vi "test_heading_calculate.vi"() -> ()   [LabVIEW 2019]
panel:
  out "new picture":picture
  out "웨이브폼 차트":dbl(graph)
  out "숫자형":i32
  in  "dt":u32=100
  in  "정지":bool
  out "UTM graph":cluster{"X":dbl, "Y":dbl}[](graph)=[{"X"=3513.14928, "Y"=12901.22133}, {"X"=3513.14928, "Y"=12901.22136}, {"X"=3513.14928, "Y"=12901.22138}, {"X"=3513.14928, "Y"=12901.2214}, {"X"=3513.14928, "Y"=12901.22142}, {"X"=3513.14928, "Y"=12901.22144}, {"X"=3513.14928, "Y"=12901.22146}, {"X"=3513.14928, "Y"=12901.22149}, {"X"=3513.14928, "Y"=12901.2215}, {"X"=3513.14926, "Y"=12901.22148}, {"X"=3513.14917, "Y"=12901.22128}, {"X"=3513.14898, "Y"=12901.22091}, {"X"=3513.14873, "Y"=12901.22045}, {"X"=3513.14844, "Y"=12901.21994}, {"X"=3513.1481, "Y"=12901.21938}, {"X"=3513.14771, "Y"=12901.21876}, {"X"=3513.14726, "Y"=12901.21808}, {"X"=3513.14671, "Y"=12901.21736}, {"X"=3513.14601, "Y"=12901.21655}, {"X"=3513.14519, "Y"=12901.21573}, {"X"=3513.14431, "Y"=12901.21489}, {"X"=3513.14358, "Y"=12901.21391}, {"X"=3513.14334, "Y"=12901.21266}, {"X"=3513.14367, "Y"=12901.21139}, {"X"=3513.14447, "Y"=12901.21041}, {"X"=3513.14553, "Y"=12901.20996}, {"X"=3513.14662, "Y"=12901.21019}, {"X"=3513.14749, "Y"=12901.21113}, {"X"=3513.14818, "Y"=12901.21232}, {"X"=3513.14884, "Y"=12901.21355}, {"X"=3513.14951, "Y"=12901.21476}, {"X"=3513.15018, "Y"=12901.21596}, {"X"=3513.15082, "Y"=12901.21716}, {"X"=3513.15145, "Y"=12901.21839}, {"X"=3513.15204, "Y"=12901.2196}, {"X"=3513.15259, "Y"=12901.22082}, {"X"=3513.15311, "Y"=12901.22201}, {"X"=3513.15351, "Y"=12901.22323}, {"X"=3513.15362, "Y"=12901.2244}, {"X"=3513.15327, "Y"=12901.22551}, {"X"=3513.15267, "Y"=12901.22636}, {"X"=3513.15188, "Y"=12901.22666}, {"X"=3513.1512, "Y"=12901.22646}, {"X"=3513.15083, "Y"=12901.22616}, {"X"=3513.15066, "Y"=12901.22594}, {"X"=3513.15061, "Y"=12901.22585}, {"X"=3513.1506, "Y"=12901.22584}, {"X"=3513.15059, "Y"=12901.22582}, {"X"=3513.15058, "Y"=12901.22581}, {"X"=3513.15058, "Y"=12901.22579}, {"X"=3513.15057, "Y"=12901.22578}, {"X"=3513.15056, "Y"=12901.22576}, {"X"=3513.15055, "Y"=12901.22575}, {"X"=3513.15054, "Y"=12901.22574}, {"X"=3513.15049, "Y"=12901.22566}, {"X"=3513.15025, "Y"=12901.22535}, {"X"=3513.1499, "Y"=12901.22478}, {"X"=3513.14967, "Y"=12901.22409}, {"X"=3513.1495, "Y"=12901.2233}, {"X"=3513.14938, "Y"=12901.22261}, {"X"=3513.14931, "Y"=12901.22222}, {"X"=3513.14927, "Y"=12901.22207}, {"X"=3513.14921, "Y"=12901.22178}, {"X"=3513.14909, "Y"=12901.22138}, {"X"=3513.14896, "Y"=12901.22104}, {"X"=3513.14895, "Y"=12901.22105}, {"X"=3513.14896, "Y"=12901.22107}, {"X"=3513.14897, "Y"=12901.22113}, {"X"=3513.14897, "Y"=12901.22113}, {"X"=3513.14897, "Y"=12901.22113}, {"X"=3513.14897, "Y"=12901.22113}, {"X"=3513.14897, "Y"=12901.22113}, {"X"=3513.14897, "Y"=12901.22112}, {"X"=3513.14897, "Y"=12901.22112}, {"X"=3513.14897, "Y"=12901.22113}, {"X"=3513.14897, "Y"=12901.22113}, {"X"=3513.14897, "Y"=12901.22113}, {"X"=3513.14897, "Y"=12901.22113}, {"X"=3513.14897, "Y"=12901.22113}, {"X"=3513.14901, "Y"=12901.2212}, {"X"=3513.14912, "Y"=12901.22153}, {"X"=3513.14922, "Y"=12901.22179}, {"X"=3513.14932, "Y"=12901.22207}, {"X"=3513.14948, "Y"=12901.2225}, {"X"=3513.1497, "Y"=12901.2231}, {"X"=3513.14982, "Y"=12901.2234}, {"X"=3513.14982, "Y"=12901.22341}, {"X"=3513.14982, "Y"=12901.22341}, {"X"=3513.14982, "Y"=12901.22341}, {"X"=3513.14982, "Y"=12901.22341}, {"X"=3513.14972, "Y"=12901.22313}, {"X"=3513.14946, "Y"=12901.22247}, {"X"=3513.14921, "Y"=12901.22185}, {"X"=3513.14908, "Y"=12901.22157}, {"X"=3513.14901, "Y"=12901.22139}, {"X"=3513.14897, "Y"=12901.2213}, {"X"=3513.14896, "Y"=12901.22125}, {"X"=3513.14891, "Y"=12901.22114}, {"X"=3513.14891, "Y"=12901.22114}, {"X"=3513.14891, "Y"=12901.22114}, {"X"=3513.14891, "Y"=12901.22114}, {"X"=3513.14891, "Y"=12901.22114}, {"X"=3513.14891, "Y"=12901.22114}, {"X"=3513.14891, "Y"=12901.22114}, {"X"=3513.14891, "Y"=12901.22114}, {"X"=3513.1489, "Y"=12901.22114}, {"X"=3513.14891, "Y"=12901.22114}, {"X"=3513.14891, "Y"=12901.22114}, {"X"=3513.14891, "Y"=12901.22114}, {"X"=3513.14891, "Y"=12901.22114}, {"X"=3513.14891, "Y"=12901.22113}, {"X"=3513.1489, "Y"=12901.22114}, {"X"=3513.1489, "Y"=12901.22114}, {"X"=3513.1489, "Y"=12901.22113}, {"X"=3513.1489, "Y"=12901.22113}, {"X"=3513.1489, "Y"=12901.22113}, {"X"=3513.1489, "Y"=12901.22113}, {"X"=3513.1489, "Y"=12901.22113}, {"X"=3513.1489, "Y"=12901.22113}, {"X"=3513.1489, "Y"=12901.22113}, {"X"=3513.1489, "Y"=12901.22113}, {"X"=3513.1489, "Y"=12901.22113}, {"X"=3513.1489, "Y"=12901.22113}, {"X"=3513.1489, "Y"=12901.22113}, {"X"=3513.1489, "Y"=12901.22113}, {"X"=3513.1489, "Y"=12901.22113}, {"X"=3513.1489, "Y"=12901.22113}, {"X"=3513.1489, "Y"=12901.22113}, {"X"=3513.1489, "Y"=12901.22113}, {"X"=3513.1489, "Y"=12901.22113}]
  in  "UTM data":cluster{"X":dbl, "Y":dbl}[](graph)=[{"X"=3513.14928, "Y"=12901.22133}, {"X"=3513.14928, "Y"=12901.22136}, {"X"=3513.14928, "Y"=12901.22138}, {"X"=3513.14928, "Y"=12901.2214}, {"X"=3513.14928, "Y"=12901.22142}, {"X"=3513.14928, "Y"=12901.22144}, {"X"=3513.14928, "Y"=12901.22146}, {"X"=3513.14928, "Y"=12901.22149}, {"X"=3513.14928, "Y"=12901.2215}, {"X"=3513.14926, "Y"=12901.22148}, {"X"=3513.14917, "Y"=12901.22128}, {"X"=3513.14898, "Y"=12901.22091}, {"X"=3513.14873, "Y"=12901.22045}, {"X"=3513.14844, "Y"=12901.21994}, {"X"=3513.1481, "Y"=12901.21938}, {"X"=3513.14771, "Y"=12901.21876}, {"X"=3513.14726, "Y"=12901.21808}, {"X"=3513.14671, "Y"=12901.21736}, {"X"=3513.14601, "Y"=12901.21655}, {"X"=3513.14519, "Y"=12901.21573}, {"X"=3513.14431, "Y"=12901.21489}, {"X"=3513.14358, "Y"=12901.21391}, {"X"=3513.14334, "Y"=12901.21266}, {"X"=3513.14367, "Y"=12901.21139}, {"X"=3513.14447, "Y"=12901.21041}, {"X"=3513.14553, "Y"=12901.20996}, {"X"=3513.14662, "Y"=12901.21019}, {"X"=3513.14749, "Y"=12901.21113}, {"X"=3513.14818, "Y"=12901.21232}, {"X"=3513.14884, "Y"=12901.21355}, {"X"=3513.14951, "Y"=12901.21476}, {"X"=3513.15018, "Y"=12901.21596}, {"X"=3513.15082, "Y"=12901.21716}, {"X"=3513.15145, "Y"=12901.21839}, {"X"=3513.15204, "Y"=12901.2196}, {"X"=3513.15259, "Y"=12901.22082}, {"X"=3513.15311, "Y"=12901.22201}, {"X"=3513.15351, "Y"=12901.22323}, {"X"=3513.15362, "Y"=12901.2244}, {"X"=3513.15327, "Y"=12901.22551}, {"X"=3513.15267, "Y"=12901.22636}, {"X"=3513.15188, "Y"=12901.22666}, {"X"=3513.1512, "Y"=12901.22646}, {"X"=3513.15083, "Y"=12901.22616}, {"X"=3513.15066, "Y"=12901.22594}, {"X"=3513.15061, "Y"=12901.22585}, {"X"=3513.1506, "Y"=12901.22584}, {"X"=3513.15059, "Y"=12901.22582}, {"X"=3513.15058, "Y"=12901.22581}, {"X"=3513.15058, "Y"=12901.22579}, {"X"=3513.15057, "Y"=12901.22578}, {"X"=3513.15056, "Y"=12901.22576}, {"X"=3513.15055, "Y"=12901.22575}, {"X"=3513.15054, "Y"=12901.22574}, {"X"=3513.15049, "Y"=12901.22566}, {"X"=3513.15025, "Y"=12901.22535}, {"X"=3513.1499, "Y"=12901.22478}, {"X"=3513.14967, "Y"=12901.22409}, {"X"=3513.1495, "Y"=12901.2233}, {"X"=3513.14938, "Y"=12901.22261}, {"X"=3513.14931, "Y"=12901.22222}, {"X"=3513.14927, "Y"=12901.22207}, {"X"=3513.14921, "Y"=12901.22178}, {"X"=3513.14909, "Y"=12901.22138}, {"X"=3513.14896, "Y"=12901.22104}, {"X"=3513.14895, "Y"=12901.22105}, {"X"=3513.14896, "Y"=12901.22107}, {"X"=3513.14897, "Y"=12901.22113}, {"X"=3513.14897, "Y"=12901.22113}, {"X"=3513.14897, "Y"=12901.22113}, {"X"=3513.14897, "Y"=12901.22113}, {"X"=3513.14897, "Y"=12901.22113}, {"X"=3513.14897, "Y"=12901.22112}, {"X"=3513.14897, "Y"=12901.22112}, {"X"=3513.14897, "Y"=12901.22113}, {"X"=3513.14897, "Y"=12901.22113}, {"X"=3513.14897, "Y"=12901.22113}, {"X"=3513.14897, "Y"=12901.22113}, {"X"=3513.14897, "Y"=12901.22113}, {"X"=3513.14901, "Y"=12901.2212}, {"X"=3513.14912, "Y"=12901.22153}, {"X"=3513.14922, "Y"=12901.22179}, {"X"=3513.14932, "Y"=12901.22207}, {"X"=3513.14948, "Y"=12901.2225}, {"X"=3513.1497, "Y"=12901.2231}, {"X"=3513.14982, "Y"=12901.2234}, {"X"=3513.14982, "Y"=12901.22341}, {"X"=3513.14982, "Y"=12901.22341}, {"X"=3513.14982, "Y"=12901.22341}, {"X"=3513.14982, "Y"=12901.22341}, {"X"=3513.14972, "Y"=12901.22313}, {"X"=3513.14946, "Y"=12901.22247}, {"X"=3513.14921, "Y"=12901.22185}, {"X"=3513.14908, "Y"=12901.22157}, {"X"=3513.14901, "Y"=12901.22139}, {"X"=3513.14897, "Y"=12901.2213}, {"X"=3513.14896, "Y"=12901.22125}, {"X"=3513.14891, "Y"=12901.22114}, {"X"=3513.14891, "Y"=12901.22114}, {"X"=3513.14891, "Y"=12901.22114}, {"X"=3513.14891, "Y"=12901.22114}, {"X"=3513.14891, "Y"=12901.22114}, {"X"=3513.14891, "Y"=12901.22114}, {"X"=3513.14891, "Y"=12901.22114}, {"X"=3513.14891, "Y"=12901.22114}, {"X"=3513.1489, "Y"=12901.22114}, {"X"=3513.14891, "Y"=12901.22114}, {"X"=3513.14891, "Y"=12901.22114}, {"X"=3513.14891, "Y"=12901.22114}, {"X"=3513.14891, "Y"=12901.22114}, {"X"=3513.14891, "Y"=12901.22113}, {"X"=3513.1489, "Y"=12901.22114}, {"X"=3513.1489, "Y"=12901.22114}, {"X"=3513.1489, "Y"=12901.22113}, {"X"=3513.1489, "Y"=12901.22113}, {"X"=3513.1489, "Y"=12901.22113}, {"X"=3513.1489, "Y"=12901.22113}, {"X"=3513.1489, "Y"=12901.22113}, {"X"=3513.1489, "Y"=12901.22113}, {"X"=3513.1489, "Y"=12901.22113}, {"X"=3513.1489, "Y"=12901.22113}, {"X"=3513.1489, "Y"=12901.22113}, {"X"=3513.1489, "Y"=12901.22113}, {"X"=3513.1489, "Y"=12901.22113}, {"X"=3513.1489, "Y"=12901.22113}, {"X"=3513.1489, "Y"=12901.22113}, {"X"=3513.1489, "Y"=12901.22113}, {"X"=3513.1489, "Y"=12901.22113}, {"X"=3513.1489, "Y"=12901.22113}, {"X"=3513.1489, "Y"=12901.22113}]
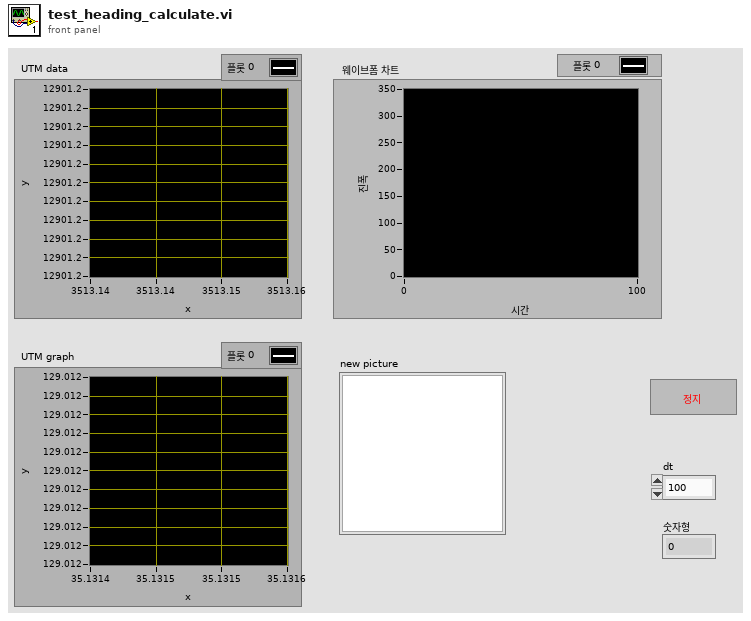
[diagram p1: front panel]
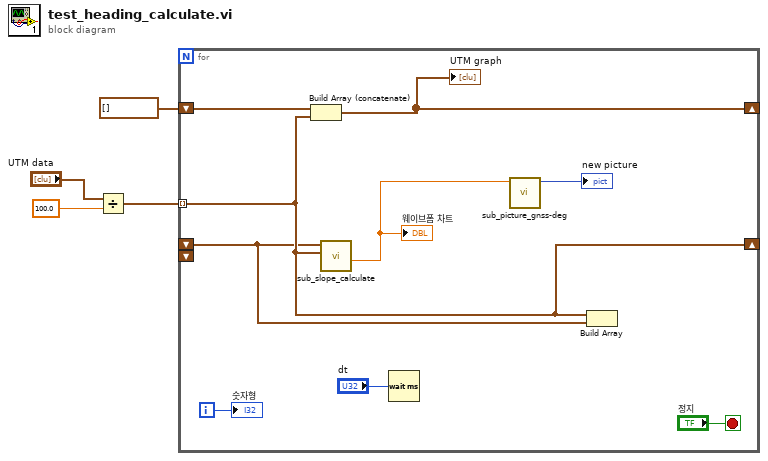
[diagram p0: block diagram]
diagram:
  n1 = Divide(x="UTM data", y=100.0) -> (x/y=w1:cluster{"X":dbl, "Y":dbl}[])
  n2 = for {
    tunnel: w1 -> [w8] mode=indexing
    shift-right: [w12] -> _
    shift-left: cluster{"X":dbl, "Y":dbl}[] [] -> [w13]
    shift-right: [w8] -> _
    shift-left: _ -> [w7]
    shift-left: _ -> [_]
    i -> [w9]
    stop <- "정지" stop-if-true
    n3 = Build Array (concatenate)(w13, w8) -> (w12:cluster{"X":dbl, "Y":dbl}[])
    "UTM graph" <- w12
    n4 = call "sub_slope_calculate.vi"("point n+1"=w8, "point n"=w7) -> ("deg_gps-base"=w6:dbl)  [unwired: 7 in, 2 out]
    "웨이브폼 차트" <- w6
    n5 = Wait (ms)(milliseconds to wait="dt") -> ()  [unwired: 1 out]
    n6 = call "sub_picture_gnss-deg.vi"("deg_gps"=w6) -> ("new picture"=→"new picture":picture)  [unwired: 10 in]
    n7 = Build Array(w8, w7) -> ()  [unwired: 1 out]
    "숫자형" <- w9
  }
